vi "SwissSPAD Live_Ready to Quit.vi"(8 "Error In":errorcluster, 9 "Flags":bool[](array[boolean]), 11 "SS2 Live Queue in":refnum<queue>) -> (0 "Error Out":errorcluster, 3 "Ready to Quit?":bool)   [LabVIEW 2021]
uses:
  SwissSPAD Live_Q [Element].ctl
  SwissSPAD Live_Q Event List.ctl
  Notebook/Notebook.lvlib
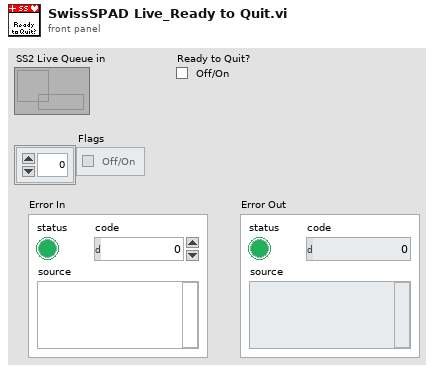
[diagram p1: front panel]
types:
  T1 = typedef "SwissSPAD Live_Q [Element].ctl" = cluster{"SwissSPAD Q Event":T2, "Data":variant}
  T2 = typedef "SwissSPAD Live_Q Event List.ctl" = enum16{"---- UI ----", "Idle", "Initialization", "Init FPGA(s)", "Init Top FPGA (deprecated)", "FPGA(s) Status", "Top FPGA Status (deprecated)", "Reset FPGA(s)", "Reset Top FPGA (deprecated)", "Refresh Display Image", "Quit", "---- DAQ ----", "Start Recording", "Start Live Acquisition", "Initialize Recording Mode", "Initialize FPGA (Live Mode)", "Get Image Set", "Get Single Image", "Update Image Display", "Stop Live Acquisition", "Stop Data Recording", "Stop Data Saving", "---- Image ----", "Copy Data to Clipboard", "Set Image Palette", "Save Displayed Image with Overlay", "Save Image Data as TIFF"}
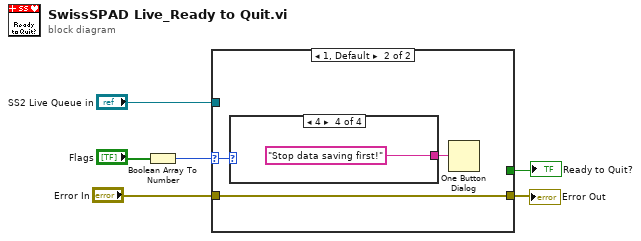
[diagram p0: block diagram]
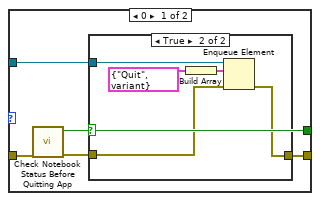
[diagram p2: hidden frame]
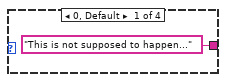
[diagram p4: hidden frame]
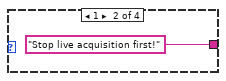
[diagram p5: hidden frame]
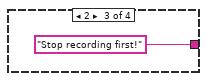
[diagram p6: hidden frame]
diagram:
  n1 = Boolean Array To Number(Boolean array="Flags") -> (number=w6:u32)
  n2 = case shown="1, Default" w6 {
    selector: w6 -> [_ w20]
    tunnel: "SS2 Live Queue in" -> [w11 _]
    tunnel: "Error In" -> [w9 w18]
    tunnel: [w10 w18] -> w2
    tunnel: [w7 _] -> w1
    frame 0 {
      n3 = call "Check Notebook Status Before Quitting App.vi"("Error In"=w9) -> ("Error Out"=w8:errorcluster, "Quit App?"=w7:bool)  [unwired: 9 in]
      n4 = case shown="True" w7 {
        tunnel: w11 -> [_ w17]
        tunnel: [w12 w14] -> w10
        tunnel: w8 -> [w12 w13]
        frame False {
        }
        frame True {
          n5 = Build Array(T1 {"SwissSPAD Q Event"=enum."Quit", "Data"=variant} ("element")) -> (w15:T1[])
          n6 = Enqueue Element(queue=w17, element=w15, error in (no error)=w13) -> (error out=w14:errorcluster)  [unwired: 1 in, 2 out]
        }
      }
    }
    frame 1, Default {
      n7 = case shown="4" w20 {
        tunnel: ["This is not supposed to happen..." ("message") "Stop live acquisition first!" ("message") "Stop recording first!" ("message") "Stop data saving first!" ("message")] -> w19
        frame 0, Default {
        }
        frame 1 {
        }
        frame 2 {
        }
        frame 4 {
        }
      }
      n8 = One Button Dialog(message=w19) -> ()  [unwired: 1 in, 1 out]
    }
  }
  "Ready to Quit?" <- w1
  "Error Out" <- w2
